vi "jsonQuery.vi"(8 "error in (no error)":errorcluster, 10 "path":string, 11 "d in":i64) -> (0 "error out":errorcluster, 1 "json type":T1, 2 "found?":bool, 3 "d out":i64)   [LabVIEW 2016, in "JSON Document.lvclass"]
uses:
  API/JSON Document Class/JSON Document.lvclass
  jsonType.ctl
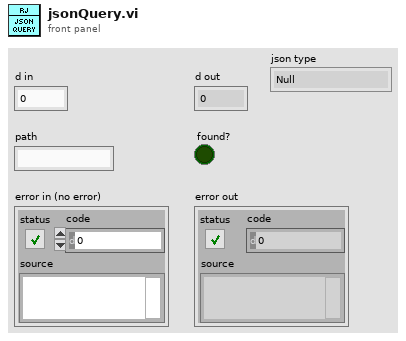
[diagram p1: front panel]
types:
  T1 = typedef "JSON Document.lvclass/jsonType.ctl" = enum16{"Null", "False", "True", "Object", "Array", "String", "Number"}
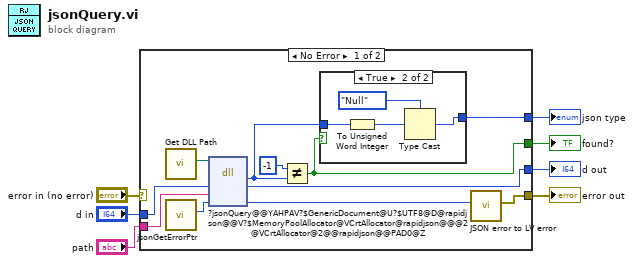
[diagram p0: block diagram]
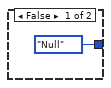
[diagram p2: hidden frame]
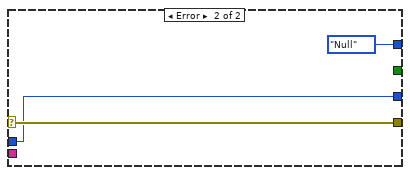
[diagram p3: hidden frame]
diagram:
  n1 = case shown="No Error" "error in (no error)" {
    selector: "error in (no error)" -> [_ w26]
    tunnel: [w11 w25] -> w7
    tunnel: "d in" -> [w16 w25]
    tunnel: "path" -> [w15 _]
    tunnel: [w13 w26] -> w4
    tunnel: [w10 _] -> w2
    tunnel: [w9 jsonType."Null" ("jsonType")] -> w1
    frame No Error {
      n2 = call "Get DLL Path.vi"() -> ("Path"=w18:path)  [unwired: 11 in]
      n3 = call "jsonGetErrorPtr.vi"() -> ("return type"=w17:i64)  [unwired: 10 in, 1 out]
      n4 = dll-call lib="C:/Users/tblair/Documents/Git Projects/LVrapidjson core/lvrjs/Debug/lvrjs.dll" fn="?jsonQuery@@YAHPAV?$GenericDocument@U?$UTF8@D@rapidjson@@V?$MemoryPoolAllocator@VCrtAllocator@rapidjson@@@2@VCrtAllocator@2@@rapidjson@@PAD0@Z"(path in=w18, "d"=w16, "path"=w15, "jsonError"=w17) -> ("return type"=w8:i32, "d"=w11:i64, "jsonError"=w14:i64)  [unwired: 3 in, 2 out]
      n5 = Not Equal?(x=-1, y=w8) -> (x != y?=w10:bool)
      n6 = case shown="True" w10 {
        tunnel: [jsonType."Null" ("jsonType") w22] -> w9
        tunnel: w8 -> [_ w21]
        frame False {
        }
        frame True {
          n7 = To Unsigned Word Integer(number=w21) -> (unsigned 16bit integer=w20:u16)
          n8 = Type Cast(type=jsonType."Null" ("jsonType"), x=w20) -> (*(type *) &x=w22:T1)
        }
      }
      n9 = call "JSON error to LV error.vi"("jsonError"=w14) -> ("error out"=w13:errorcluster)  [unwired: 10 in]
    }
    frame Error {
    }
  }
  "found?" <- w2
  "d out" <- w7
  "error out" <- w4
  "json type" <- w1
